vi "Interactive Graph Test.vi"() -> ()   [LabVIEW 2015]
uses:
  Interactive Graph/Interactive Graph.xctl
  Math VIs/LinSpace (x0-dx-npts).vi
  <vilib>/Analysis/1siggen.llb/General Gauss-Mod Sine.vi
  <vilib>/Analysis/NI_AALBase.lvlib
panel:
  out "Max":dbl
  out "Value 2":dbl
  out "Y0":dbl
  out "Value":i32
  out "Cursor":cluster{"X":dbl, "Y":dbl}
  in  "Cursor":bool
  in  "Graph":T2(xcontrol)
  in  "Dummy Data":bool
  in  "stop":bool
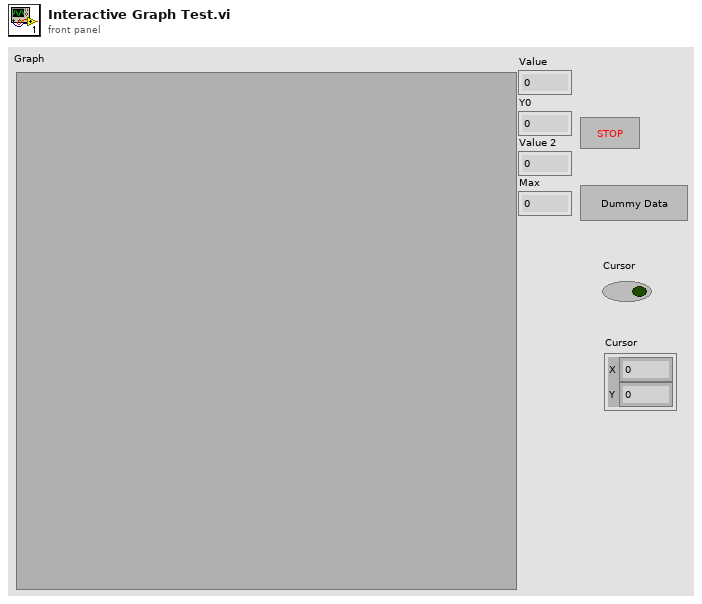
[diagram p1: front panel]
types:
  T1 = typedef "EPhysWork-Label Position.ctl" = cluster{"Index":i32, "Xoff":dbl, "Yoff":dbl}
  T2 = cluster{"plot":cluster{"X":dbl[], "Y":dbl[]}, "name":string, "Y0":dbl, "color":u32, "Style":enum16{"Normal", "Highlight", "Shadow"}, "labpos":T1, "visible":bool, "cursor":bool}[]
  T3 = typedef "Interactive Graph.xctl/Events.ctl" = cluster{"Selection":refnum<user-event>, "XRange":refnum<user-event>, "YScale":refnum<user-event>, "CursorPos":refnum<user-event>}
  T4 = cluster{"plot":cluster{"X":dbl[], "Y":dbl[]}, "name":string, "Y0":dbl, "color":u32, "Style":enum16{"Normal", "Highlight", "Shadow"}, "labpos":T1, "visible":bool, "cursor":bool}
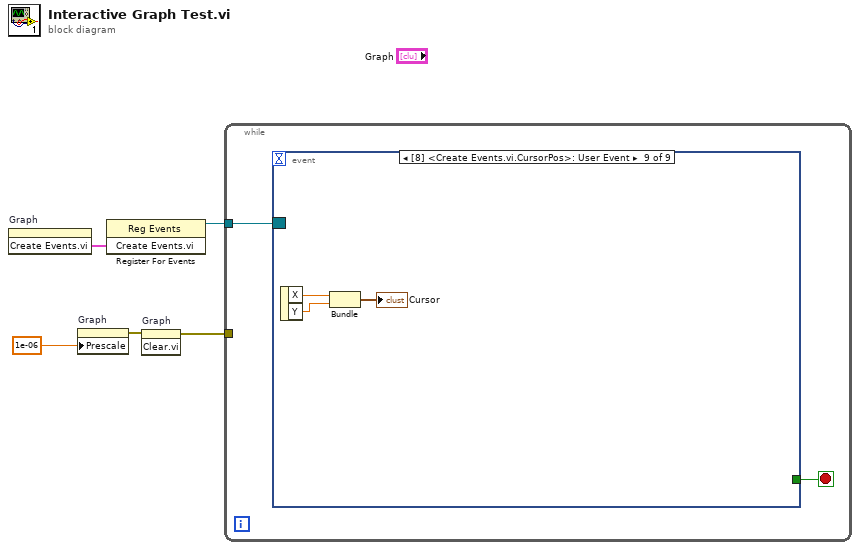
[diagram p0: block diagram]
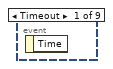
[diagram p2: hidden frame]
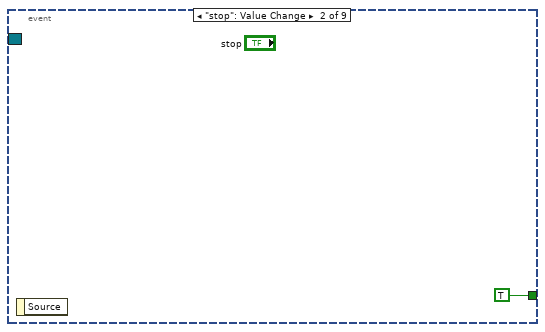
[diagram p3: hidden frame]
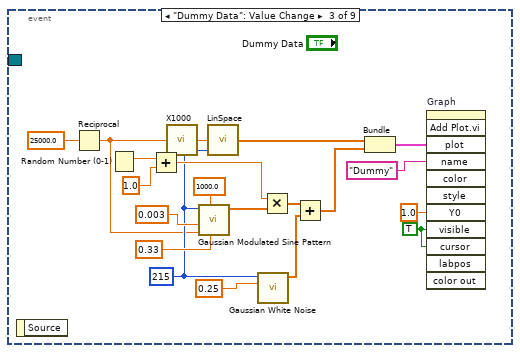
[diagram p4: hidden frame]
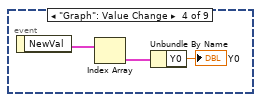
[diagram p5: hidden frame]
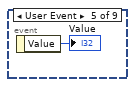
[diagram p6: hidden frame]
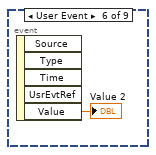
[diagram p7: hidden frame]
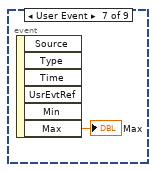
[diagram p8: hidden frame]
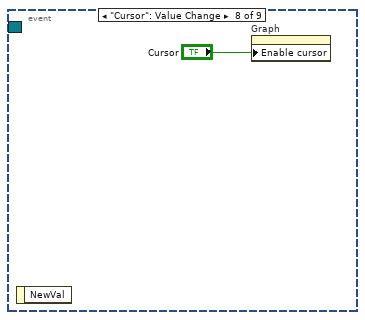
[diagram p9: hidden frame]
diagram:
  n1 = invoke on="Graph" class="Interactive Graph (strict)" method="Create Events.vi"() -> ("Create Events.vi"=w1:T3)  [unwired: 3 in, 2 out]
  n2 = property on="Graph" class="IGraph (strict)"("Prescale"=1e-06) -> (error out=w4:errorcluster)  [unwired: 2 in, 1 out]
  n3 = register-events(w1) -> (reference out=w2:refnum<event-registration>)  [unwired: 2 in, 1 out]
  n4 = invoke on="Graph" class="Interactive Graph (strict)" method="Clear.vi"(error in=w4) -> (error out=w5:errorcluster)  [unwired: 2 in, 2 out]
  n5 = while {
    tunnel: w5 -> [_]
    tunnel: w2 -> [w6]
    stop <- w7 stop-if-true
    n6 = event shown="[8] <Create Events.vi.CursorPos>: User Event" {
      selector: w6 -> [_ _ _ _ _ _ _ _ _]
      dyn-events: _ -> [_ _ _ _ _ _ _ _ _]
      timeout: _ -> [_ _ _ _ _ _ _ _ _]
      tunnel: [_ TRUE _ _ _ _ _ _ _] -> w7
      event Timeout {
        n7 = event-data() -> ()  [unwired: 1 in, 1 out]
      }
      event "stop": Value Change {
        n8 = event-data() -> ()  [unwired: 1 in, 1 out]
      }
      event "Dummy Data": Value Change {
        w9 = TRUE ("cursor")
        w17 = 215 ("samples")
        n9 = event-data() -> ()  [unwired: 1 in, 1 out]
        n10 = Reciprocal(x=25000.0 ("Fs")) -> (1/x=w16:dbl)
        n11 = Random Number (0-1)() -> (number: 0 to 1=w24:dbl)
        n12 = Add(x=w24, y=1.0) -> (x+y=w26:dbl)
        n13 = call "X1000.vi"("X"=w16) -> ("X/1000"=w11:dbl)
        n14 = call <vilib>:"Gaussian Modulated Sine Pattern.vi"("normalized bandwidth"=0.33, "center frequency (Hz)"=1000.0 ("y"), "delta t (s)"=w16, "delay (s)"=0.003, "samples"=w17) -> ("Gauss-Mod Sine Pattern"=w21:dbl[])  [unwired: 5 in, 1 out]
        n15 = call-poly "LinSpace.vi"("npts"=w17, "dx"=w11) -> ("Array"=w15:dbl[])  [unwired: 2 in, 1 out]
        n16 = call <vilib>:"Gaussian White Noise.vi"("standard deviation"=0.25, "samples"=w17) -> ("Gaussian noise pattern"=w19:dbl[])  [unwired: 8 in, 1 out]
        n17 = Multiply(x=w26, y=w21) -> (x*y=w23:dbl[])
        n18 = Add(x=w23, y=w19) -> (x+y=w14:dbl[])
        n19 = Bundle("Array"=w15, w14) -> (w13:cluster{"Array":dbl[], dbl[]})  [unwired: 1 in]
        n20 = invoke on="Graph" class="Interactive Graph (strict)" method="Add Plot.vi"("plot"=w13, "name"="Dummy", "Y0"=1.0, "visible"=w9, "cursor"=w9) -> ()  [unwired: 7 in, 12 out]
      }
      event "Graph": Value Change {
        n21 = event-data() -> ("NewVal"=w31:T2)  [unwired: 1 in]
        n22 = Index Array(array=w31) -> (element=w30:T4)  [unwired: 1 in]
        n23 = Unbundle By Name(w30) -> ("Y0"=→"Y0":dbl)
      }
      event User Event {
        n24 = event-data() -> ("Value"=→"Value":i32)  [unwired: 1 in]
      }
      event User Event {
        n25 = event-data() -> ("Value"=→"Value 2":dbl)  [unwired: 1 in, 4 out]
      }
      event User Event {
        n26 = event-data() -> ("Max"=→"Max":dbl)  [unwired: 1 in, 5 out]
      }
      event "Cursor": Value Change {
        n27 = event-data() -> ()  [unwired: 1 in, 1 out]
        n28 = property on="Graph" class="IGraph (strict)"("Enable cursor"="Cursor") -> ()  [unwired: 2 in, 2 out]
      }
      event User Event {
        n29 = event-data() -> ("X"=w38:dbl, "Y"=w37:dbl)  [unwired: 1 in]
        n30 = Bundle("X"=w38, "Y"=w37) -> (→"Cursor":cluster{"X":dbl, "Y":dbl})  [unwired: 1 in]
      }
    }
  }
